vi "MultiTone.vi"(6 "Sampling Info":cluster{"Fs":dbl, "#s":dbl}={"Fs"=1000.0, "#s"=1000.0} {"Fs" format="%.2p"}, 9 "Signal type":T1(ring), 10 "Amplitudes":dbl[](array[numeric]), 11 "Frequences":dbl[](array[numeric])) -> (3 "Output":waveform(dbl))   [LabVIEW 2024]
uses:
  <vilib>/measure/NI_MABase.lvlib
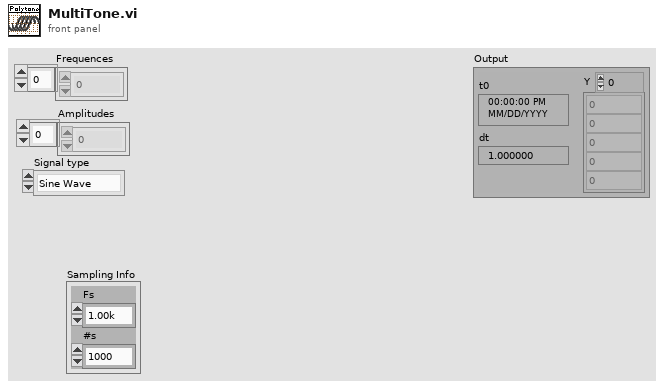
[diagram p1: front panel]
types:
  T1 = enum16{"Sine Wave", "Triangle Wave", "Square Wave", "Sawtooth Wave"}
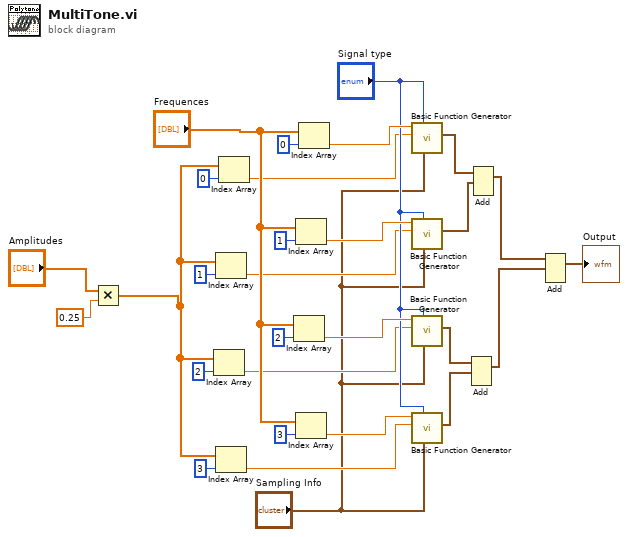
[diagram p0: block diagram]
diagram:
  n1 = Multiply(x="Amplitudes", y=0.25 ("element")) -> (x*y=w2:dbl[])
  n2 = Index Array(array=w2, index=2) -> (element=w7:dbl)
  n3 = Index Array(array=w2, index=1) -> (element=w6:dbl)
  n4 = Index Array(array=w2, index=3) -> (element=w8:dbl)
  n5 = Index Array(array=w2, index=0) -> (element=w5:dbl)
  n6 = Index Array(array="Frequences", index=2) -> (element=w20:dbl)
  n7 = Index Array(array="Frequences", index=1) -> (element=w22:dbl)
  n8 = Index Array(array="Frequences", index=3) -> (element=w19:dbl)
  n9 = Index Array(array="Frequences", index=0) -> (element=w21:dbl)
  n10 = call <vilib>:"Basic Function Generator.vi"("sampling info"="Sampling Info", "signal type"="Signal type", "amplitude"=w5, "frequency"=w21) -> ("signal out"=w29:waveform(dbl))  [unwired: 5 in, 2 out]
  n11 = call <vilib>:"Basic Function Generator.vi"("sampling info"="Sampling Info", "signal type"="Signal type", "amplitude"=w6, "frequency"=w22) -> ("signal out"=w28:waveform(dbl))  [unwired: 5 in, 2 out]
  n12 = call <vilib>:"Basic Function Generator.vi"("sampling info"="Sampling Info", "signal type"="Signal type", "amplitude"=w7, "frequency"=w20) -> ("signal out"=w27:waveform(dbl))  [unwired: 5 in, 2 out]
  n13 = call <vilib>:"Basic Function Generator.vi"("sampling info"="Sampling Info", "signal type"="Signal type", "amplitude"=w8, "frequency"=w19) -> ("signal out"=w26:waveform(dbl))  [unwired: 5 in, 2 out]
  n14 = Add(1:w26, 2:w27) -> (0:w25:waveform(dbl))  [unwired: 1 in, 1 out]
  n15 = Add(1:w28, 2:w29) -> (0:w24:waveform(dbl))  [unwired: 1 in, 1 out]
  n16 = Add(1:w25, 2:w24) -> (0:→"Output":waveform(dbl))  [unwired: 1 in, 1 out]
